vi "FTW-Container-Element-Path.vi"(0 "FTW-Container In":refnum<class "FTW-Container.lvclass">, 5 "Element Path":string[](array[string]), 11 "error in":errorcluster) -> (4 "FTW-Container Out":refnum<class "FTW-Container.lvclass">, 6 "Element Out":refnum<class "FTW-Container.lvclass">, 8 "Found":bool, 15 "error out":errorcluster)   [LabVIEW 2015, in "FTW-Container.lvclass"]
uses:
  FTW-Container.lvclass
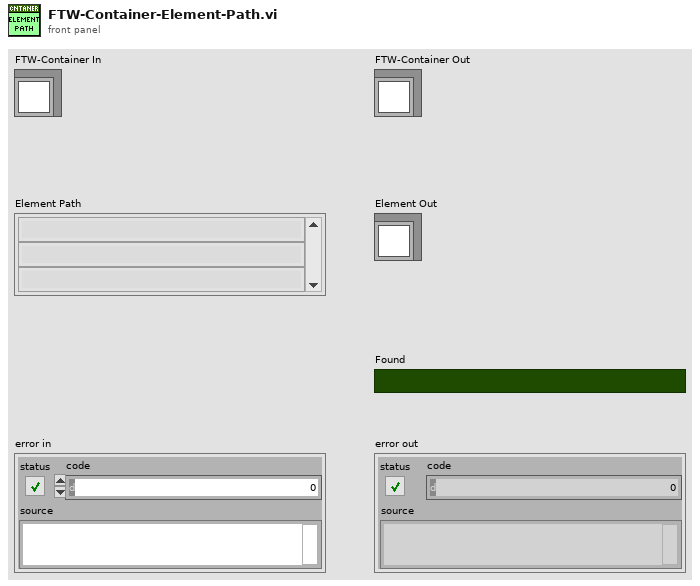
[diagram p1: front panel]
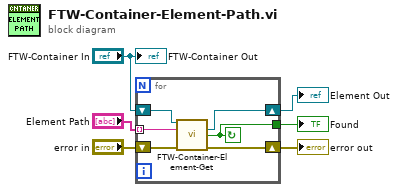
[diagram p0: block diagram]
diagram:
  n1 = for {
    tunnel: "Element Path" -> [w9] mode=indexing
    shift-right: [w10] -> w4
    shift-left: "error in" -> [w11]
    shift-right: [w8] -> w1
    shift-left: "FTW-Container In" -> [w12]
    tunnel: [w7] -> w2
    stop <- w7 continue-if-true
    n2 = call "FTW-Container-Element-Get.vi"("FTW-Container In"=w12, "Element Name"=w9, "error in"=w11) -> ("Element Out"=w8:refnum<class "FTW-Container.lvclass">, "Found"=w7:bool, "error out"=w10:errorcluster)  [unwired: 9 in, 1 out]
  }
  "error out" <- w4
  "Element Out" <- w1
  "Found" <- w2
  "FTW-Container Out" <- "FTW-Container In"
